vi "Main Host MSS test.vi"() -> ()   [LabVIEW 2023]
uses:
  <vilib>/ni/Actors/Network Endpoint Actors/Protocols/Network Stream Strategy/Network Stream Initiator/Network Stream Initiator.lvclass
  MSS/MSS Host Actor/MSS Host Actor.lvclass
  <vilib>/ActorFramework/Actor/Actor.lvclass
panel:
  in  "Remote Address":string="169.254.205.87"
  in  "Address":string="169.254.205.1"
  out "error out":errorcluster
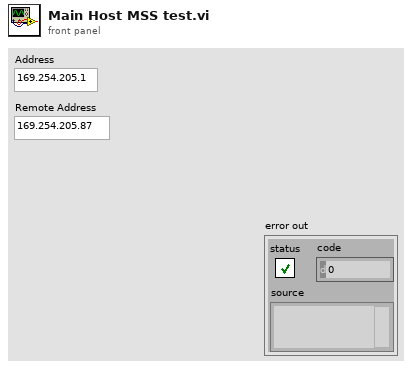
[diagram p1: front panel]
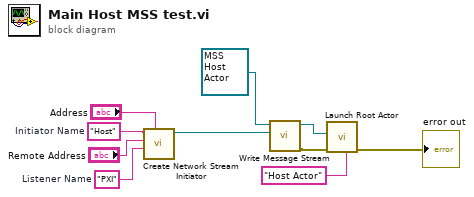
[diagram p0: block diagram]
diagram:
  w2 = "PXI"  # Listener Name
  w10 = "Host"  # Initiator Name
  n1 = call <vilib>:"Create Network Stream Initiator.vi"("Local Address"="Address", "Remote Name"=w2, "Remote Address"="Remote Address", "Name"=w10) -> ("Network Stream Initiator out"=w7:refnum<class "Network Stream Initiator.lvclass">)  [unwired: 7 in]
  n2 = call "Write Message Stream.vi"("Message Stream.lvclass"=w7, "MSS Host Actor in"=refnum<class "MSS Host Actor.lvclass"> refnum ("MSS Host Actor.lvlib:MSS Host Actor.lvclass")) -> ("error out"=w6:errorcluster, "MSS Host Actor out"=w4:refnum<class "MSS Host Actor.lvclass">)  [unwired: 8 in]
  n3 = call <vilib>:"Launch Root Actor.vi"("Debug Alias"="Host Actor", "error in (no error)"=w6, "Actor"=w4) -> ("error out"=→"error out":errorcluster)  [unwired: 7 in, 1 out]
